vi "Read HttpRequestMessage.vi"(8 "error in (no error)":errorcluster, 11 "HttpResponseMessage in":refnum<class "HttpResponseMessage.lvclass">) -> (0 "error out":errorcluster, 2 "LabVIEWHTTPClient_NET.lvlib:HttpRequestMessage.lvclass":refnum<class "HttpRequestMessage.lvclass">, 3 "HttpResponseMessage out":refnum<class "HttpResponseMessage.lvclass">)   [LabVIEW 2018, in "HttpClient_NET.lvlib" / "HttpResponseMessage.lvclass"]
uses:
  HttpResponseMessage.lvclass
  HttpRequestMessage/HttpRequestMessage.lvclass
  HttpResponseMessage.lvclass/HttpResponseMessage.ctl
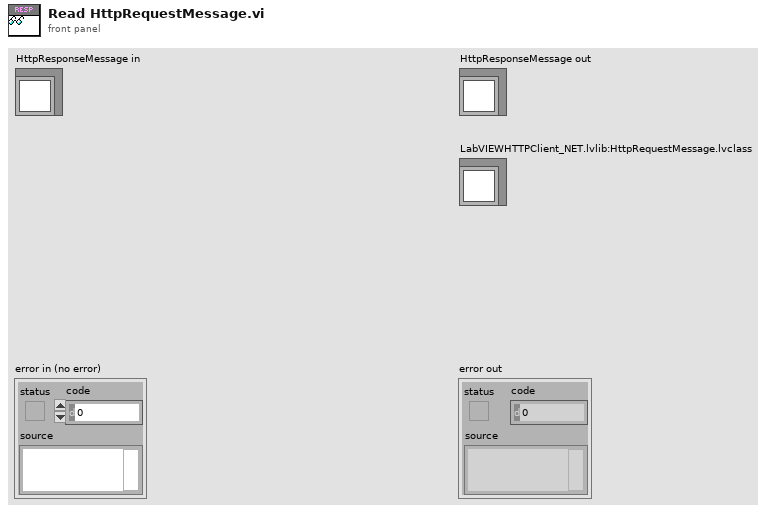
[diagram p1: front panel]
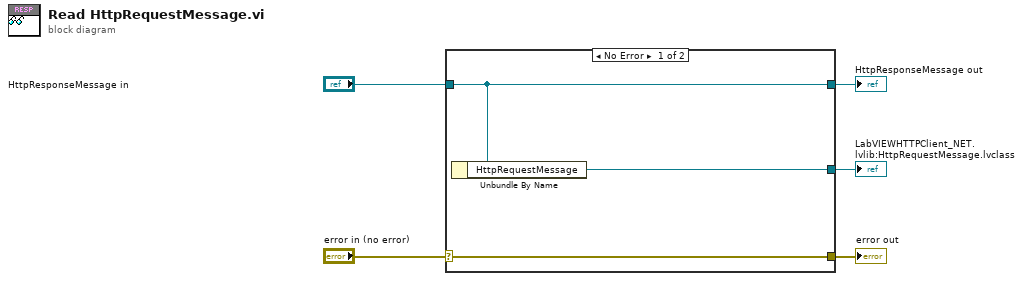
[diagram p0: block diagram]
diagram:
  n1 = case shown="No Error" "error in (no error)" {
    selector: "error in (no error)" -> [w8 w9]
    tunnel: [w8 w9] -> w4
    tunnel: [w7 w10] -> w2
    tunnel: "HttpResponseMessage in" -> [w7 w10]
    tunnel: [w6 _] -> w1
    frame No Error {
      n2 = Unbundle By Name(w7) -> ("HttpRequestMessage"=w6:refnum<class "HttpRequestMessage.lvclass">)
    }
    frame Error {
    }
  }
  "error out" <- w4
  "HttpResponseMessage out" <- w2
  "LabVIEWHTTPClient_NET.lvlib:HttpRequestMessage.lvclass" <- w1
